vi "Equip-Read config.vi"(0 "AO Map":T1, 5 "AI Map":T1, 7 "config name":string="Connections", 9 "slot ctl refs":refnum<vi>[](array[refnum]), 11 "error in (no error)":errorcluster) -> (4 "Hide unused?":bool, 15 "error out":errorcluster)   [LabVIEW 2020]
uses:
  Type Defs/Output sources.ctl
  Type Defs/Input sources.ctl
  Type Defs/PXISlot XControl/PXISlot.xctl
  Utility VIs/Array Manipulation VIs/Array-Dimensions (2D).vi
  <vilib>/Utility/config.llb/Read Key (I32).vi
  <vilib>/Utility/config.llb/Read Key (Boolean).vi
  <vilib>/Utility/config.llb/NI_LVConfig.lvlib
panel:
  in  "Input sources":T2 items=["--unused--", "Probe Mic Right", "Probe Mic Left", "Cal Mic", "ABR", "CAP Right", "CAP Left", "Startle piezo", "Temperature", "Heart rate", "Accelerometer", "Startle piezo 2"]
  in  "Output sources":T3 items=["--unused--", "Right primary", "Right secondary", "Left primary", "Left secondary", "Shocks", "Startle", "Background", "Shaker", "Blue laser"]
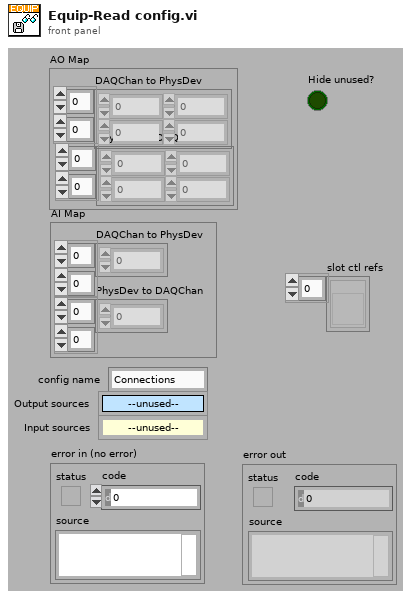
[diagram p1: front panel]
types:
  T1 = cluster{"DAQChan to PhysDev":i32[][], "PhysDev to DAQChan":i32[][]}
  T2 = typedef "Input sources.ctl" = u16
  T3 = typedef "Output sources.ctl" = u16
  T4 = typedef "NI_LVConfig.lvlib/Config Data RefNum.ctl" = refnum<k1>
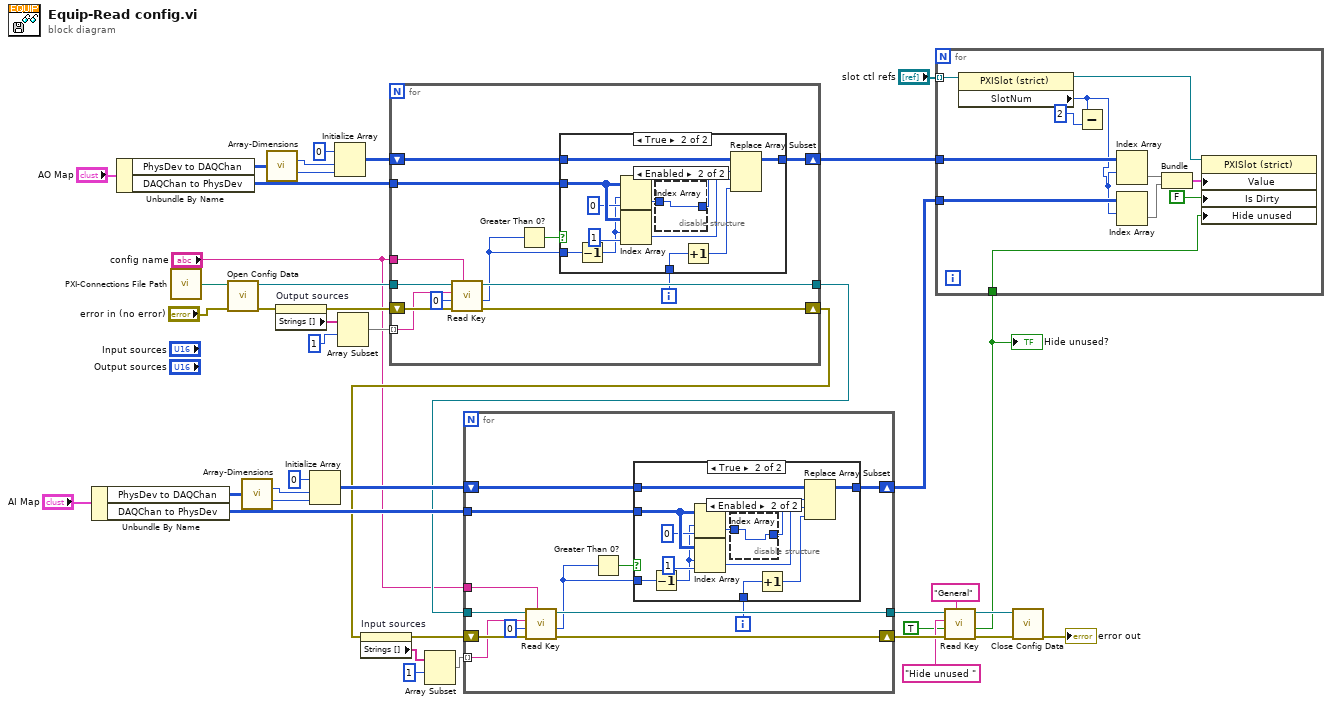
[diagram p0: block diagram]
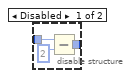
[diagram p3: hidden frame]
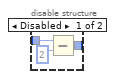
[diagram p5: hidden frame]
diagram:
  n1 = Unbundle By Name("AI Map") -> ("PhysDev to DAQChan"=w24:i32[][], "DAQChan to PhysDev"=w18:i32[][])
  n2 = Unbundle By Name("AO Map") -> ("PhysDev to DAQChan"=w31:i32[][], "DAQChan to PhysDev"=w33:i32[][])
  n3 = call "PXI-Connections File Path.vi"() -> ("Path"=w1:path)  [unwired: 1 in]
  n4 = call <vilib>:"Open Config Data.vi"("error in (no error)"="error in (no error)", "configuration file path"=w1) -> ("error out"=w40:errorcluster, "refnum"=w35:T4)  [unwired: 7 in, 1 out]
  n5 = call-poly "Array-Dimensions.vi"("2D Array"=w24) -> ("# rows"=w23:i32, "# columns"=w22:i32)  [unwired: 13 in]
  n6 = call-poly "Array-Dimensions.vi"("2D Array"=w31) -> ("# rows"=w30:i32, "# columns"=w29:i32)  [unwired: 13 in]
  n7 = property on="Output sources" class="Ring (strict)"(error in=w40) -> (error out=w36:errorcluster, "Strings []"=w39:string[])  [unwired: 1 in, 1 out]
  n8 = Initialize Array(0 ("element"), w23, w22) -> (w19:i32[][])
  n9 = Initialize Array(0 ("element"), w30, w29) -> (w27:i32[][])
  n10 = Array Subset(array=w39, index=1) -> (w37:string[])  [unwired: 1 in]
  n11 = for {
    tunnel: w37 -> [w51] mode=indexing
    tunnel: w35 -> [w53]
    tunnel: "config name" -> [w52]
    tunnel: w33 -> [w49]
    shift-right: [w47] -> w25
    shift-left: w27 -> [w48]
    tunnel: [w46] -> w15
    shift-right: [w45] -> w16
    shift-left: w36 -> [w54]
    i -> [w44]
    n12 = call-poly <vilib>:"Read Key.vi"("section"=w52, "error in (no error)"=w54, "default value"=0, "key"=w51, "refnum"=w53) -> ("error out"=w45:errorcluster, "value"=w42:i32, "refnum out"=w46:T4)  [unwired: 3 in, 1 out]
    n13 = Greater Than 0?(x=w42) -> (x > 0?=w43:bool)
    n14 = case shown="True" w43 {
      tunnel: w49 -> [_ w67]
      tunnel: w48 -> [w55 w66]
      tunnel: [w55 w65] -> w47
      tunnel: w42 -> [_ w59]
      tunnel: w44 -> [_ w58]
      frame False {
      }
      frame True {
        n15 = Decrement(x=w59) -> (x-1=w56:i32)
        n16 = Index Array(array=w67, index (row)=w56, index (col)=0 ("length")) -> (element=w60:i32)
        n17 = Index Array(array=w67, index (row)=w56, index (col)=1 ("length")) -> (element=w62:i32)
        n18 = disable-structure shown="Enabled" {
          disable-tunnel: [w70 w71] -> w61
          disable-tunnel: w60 -> [w69 w71]
          frame Disabled {
            n19 = Subtract(x=w69, y=2) -> (x-y=w70:i32)
          }
          frame Enabled {
          }
        }
        n20 = Increment(x=w58) -> (x+1=w57:i32)
        n21 = Replace Array Subset(array=w66, new element=w57, index (row)=w61, index (col)=w62) -> (w65:i32[][])
      }
    }
  }
  n22 = property on="Input sources" class="Ring (strict)"(error in=w16) -> (error out=w17:errorcluster, "Strings []"=w13:string[])  [unwired: 1 in, 1 out]
  n23 = Array Subset(array=w13, index=1) -> (w12:string[])  [unwired: 1 in]
  n24 = for {
    tunnel: w12 -> [w81] mode=indexing
    tunnel: w15 -> [w83]
    tunnel: "config name" -> [w82]
    tunnel: w18 -> [w79]
    shift-right: [w77] -> w14
    shift-left: w19 -> [w78]
    tunnel: [w76] -> w7
    shift-right: [w75] -> w10
    shift-left: w17 -> [w84]
    i -> [w74]
    n25 = call-poly <vilib>:"Read Key.vi"("section"=w82, "error in (no error)"=w84, "default value"=0, "key"=w81, "refnum"=w83) -> ("error out"=w75:errorcluster, "value"=w72:i32, "refnum out"=w76:T4)  [unwired: 3 in, 1 out]
    n26 = Greater Than 0?(x=w72) -> (x > 0?=w73:bool)
    n27 = case shown="True" w73 {
      tunnel: w79 -> [_ w97]
      tunnel: w78 -> [w85 w96]
      tunnel: [w85 w95] -> w77
      tunnel: w72 -> [_ w89]
      tunnel: w74 -> [_ w88]
      frame False {
      }
      frame True {
        n28 = Decrement(x=w89) -> (x-1=w86:i32)
        n29 = Index Array(array=w97, index (row)=w86, index (col)=0 ("length")) -> (element=w90:i32)
        n30 = Index Array(array=w97, index (row)=w86, index (col)=1 ("length")) -> (element=w92:i32)
        n31 = disable-structure shown="Enabled" {
          disable-tunnel: [w100 w101] -> w91
          disable-tunnel: w90 -> [w99 w101]
          frame Disabled {
            n32 = Subtract(x=w99, y=2) -> (x-y=w100:i32)
          }
          frame Enabled {
          }
        }
        n33 = Increment(x=w88) -> (x+1=w87:i32)
        n34 = Replace Array Subset(array=w96, new element=w87, index (row)=w91, index (col)=w92) -> (w95:i32[][])
      }
    }
  }
  n35 = call-poly <vilib>:"Read Key.vi"("section"="General", "error in (no error)"=w10, "default value"=TRUE, "key"="Hide unused ", "refnum"=w7) -> ("error out"=w9:errorcluster, "value"=w3:bool, "refnum out"=w8:T4)  [unwired: 3 in, 1 out]
  "Hide unused?" <- w3
  n36 = for {
    tunnel: "slot ctl refs" -> [w111] mode=indexing
    tunnel: w25 -> [w106]
    tunnel: w14 -> [w109]
    tunnel: w3 -> [w103]
    n37 = property class="PXISlot (strict)"(reference=w111) -> (reference out=w110:refnum<vi>, "SlotNum"=w102:i32)  [unwired: 1 in, 1 out]
    n38 = Subtract(x=w102, y=2) -> ()  [unwired: 1 out]
    n39 = Index Array(array=w106, index (row)=w102) -> (element=w105:i32[])  [unwired: 1 in]
    n40 = Index Array(array=w109, index (row)=w102) -> (element=w107:i32[])  [unwired: 1 in]
    n41 = Bundle(w105, w107) -> (w112:cluster{i32[], i32[]})  [unwired: 1 in]
    n42 = property class="PXISlot (strict)"(reference=w110, "Value"=w112, "Is Dirty"=FALSE, "Hide unused"=w103) -> ()  [unwired: 1 in, 2 out]
  }
  n43 = call <vilib>:"Close Config Data.vi"("error in (no error)"=w9, "refnum"=w8) -> ("error out"=→"error out":errorcluster)  [unwired: 8 in, 1 out]
